vi "Enable-Disable UI by Parameter Sweep.vi"() -> (3 "Controls refs to enable/disable":refnum<vi>[](array[refnum]))   [LabVIEW 2017]
uses:
  Global Variables/gl_UI Ctrl Refs.vi
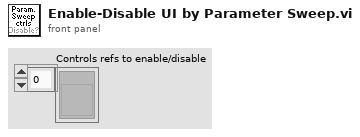
[diagram p1: front panel]
types:
  T1 = typedef "UI ctrl refs cluster.ctl" = cluster{"Top level VI path":path, "Top level VI ref":refnum<vi>, "User menu ref":refnum<k9>, "Sub Panel control":refnum<vi>, "Imaging Param Tab":refnum<vi>, "Occurrence-Start drivers":refnum<k4>, "Occurrence-Speed logging initialised":refnum<k4>, "Occurrence-XYZ stage initialised":refnum<k4>, "Exit button":refnum<vi>, "Status ind":refnum<vi>, "Set as origin":refnum<vi>, "Speed Logging":refnum<vi>, "Time Lapse":refnum<vi>, "Live Imaging":refnum<vi>, "AOL Z Stack":refnum<vi>, "Motor Z Stack":refnum<vi>, "Funct Acq button":refnum<vi>, "Hard Shutter":refnum<vi>, "Virtual Shutter":refnum<vi>, "Laser Power":refnum<vi>, "AOL Mode":refnum<vi>, "Frame Size":refnum<vi>, "Field of View":refnum<vi>, "Dwell Time":refnum<vi>, "Zoom":refnum<vi>, "AOL Z":refnum<vi>, "Objective":refnum<vi>, "Axis":refnum<vi>, "Paths & Names":refnum<vi>, "Experiment folder path (ind.)":refnum<vi>, "Last State (Ind.)":refnum<vi>, "Averages":refnum<vi>, "Angle (degrees)":refnum<vi>, "X centre":refnum<vi>, "Y centre":refnum<vi>, "Plane Mode":refnum<vi>, "# Planes":refnum<vi>, "Z Start":refnum<vi>, "Z Stop":refnum<vi>, "Z Step":refnum<vi>, "PMT 1":refnum<vi>, "PMT 2":refnum<vi>, "Stage XYZ Position":refnum<vi>, "Pockels@Z Start":refnum<vi>, "Pockels@Z Stop":refnum<vi>, "Obtain Z Start":refnum<vi>, "Obtain Z Stop":refnum<vi>, "Live stim.trig.period":refnum<vi>, "Live stim.trig.enable":refnum<vi>, "Movement Correction":refnum<vi>, "Load Reference Image":refnum<vi>, "XY Stage Move":refnum<vi>, "MovCor Cluster":refnum<vi>, "RefDAQParam":refnum<vi>, "Funct. Acq. Pockels Modulation":refnum<vi>, "Ref Laser Power":refnum<vi>, "Enable Video Recording":refnum<vi>, "Video Record-Live Imaging":refnum<vi>, "Video Record-Funct acq":refnum<vi>, "Reference Source":refnum<vi>, "AOL Z-stack Chirps Ready (ind)":refnum<vi>, "Target time between mov.cor. ref triggers (ms)":refnum<vi>, "Funct. Acq. Ref frame save":refnum<vi>, "Tracking button":refnum<vi>, "Show ref plots window":refnum<vi>, "Center freq ind (nm)":refnum<vi>, "Pickup mode (ind)":refnum<vi>, "Logging queue (ind)":refnum<vi>, "Back aperture power (ind.)":refnum<vi>, "Power after objective (ind.)":refnum<vi>, "Switch user":refnum<vi>, "Ls1 Conn. Status":refnum<vi>, "Ls1Tuning Status":refnum<vi>, "Ls1 Faults":refnum<vi>, "Ls1 Connection":refnum<vi>, "Ls1 Mode":refnum<vi>, "Ls1 POWER [mW]":refnum<vi>, "Ls1Shutter":refnum<vi>, "Ls1 Wavelength":refnum<vi>, "Ls1 Note":refnum<vi>, "Ls1 Confirm Wav":refnum<vi>, "Ls1 PreChrp Prism1":refnum<vi>, "Ls1 PreChrp Prism2":refnum<vi>, "Ls1 wav top Ind":refnum<vi>, "Ls1 power top Ind":refnum<vi>, "Ls1 Pump peak Hold":refnum<vi>, "Ls1 Status Ind":refnum<vi>, "Ls1 wav cancel":refnum<vi>, "Experiment Type":refnum<vi>, "Biology Information":refnum<vi>, "Camera recording status":refnum<vi>, "Start Sweep":refnum<vi>, "# Sw. Planes":refnum<vi>}
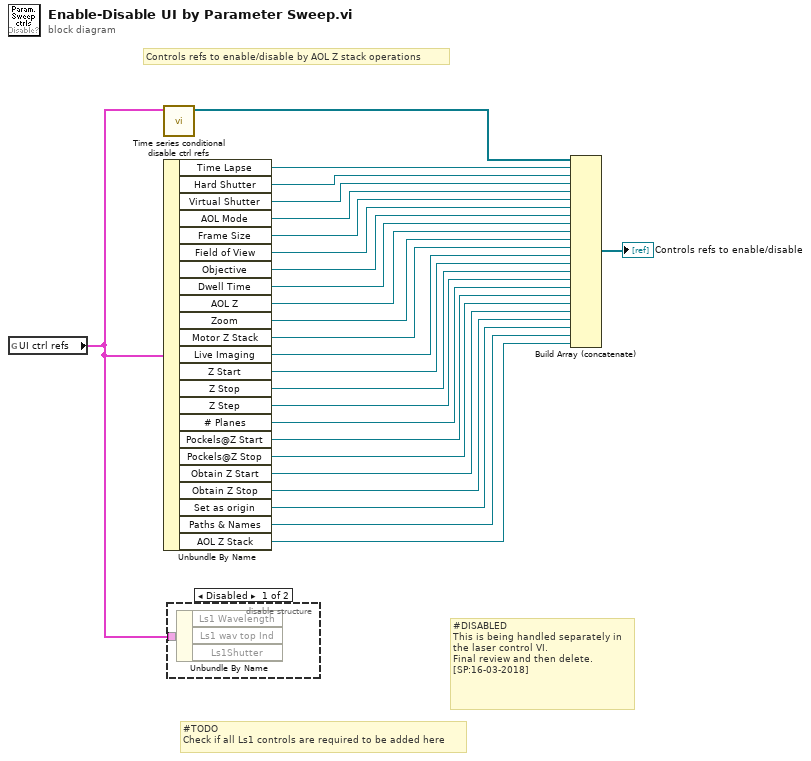
[diagram p0: block diagram]
diagram:
  # "#DISABLED\nThis is being handled separately in\nthe laser control VI.\nFinal review and then delete.\n[SP:16-03-2018]"
  # "#TODO\nCheck if all Ls1 controls are required to be added here"
  # "Controls refs to enable/disable by AOL Z stack operations"
  n1 = global read "gl_UI Ctrl Refs.vi" "UI ctrl refs"() -> (w2:T1)
  n2 = call "Time series conditional disable ctrl refs.vi"("UI ctrl refs"=w2) -> ("Ctrl refs"=w13:refnum<vi>[])  [unwired: 10 in]
  n3 = Unbundle By Name(w2) -> ("Time Lapse"=w26:refnum<vi>, "Hard Shutter"=w22:refnum<vi>, "Virtual Shutter"=w21:refnum<vi>, "AOL Mode"=w20:refnum<vi>, "Frame Size"=w19:refnum<vi>, "Field of View"=w18:refnum<vi>, "Objective"=w17:refnum<vi>, "Dwell Time"=w16:refnum<vi>, "AOL Z"=w15:refnum<vi>, "Zoom"=w14:refnum<vi>, "Motor Z Stack"=w24:refnum<vi>, "Live Imaging"=w25:refnum<vi>, "Z Start"=w12:refnum<vi>, "Z Stop"=w11:refnum<vi>, "Z Step"=w10:refnum<vi>, "# Planes"=w9:refnum<vi>, "Pockels@Z Start"=w8:refnum<vi>, "Pockels@Z Stop"=w7:refnum<vi>, "Obtain Z Start"=w6:refnum<vi>, "Obtain Z Stop"=w5:refnum<vi>, "Set as origin"=w4:refnum<vi>, "Paths & Names"=w3:refnum<vi>, "AOL Z Stack"=w1:refnum<vi>)
  n4 = disable-structure shown="Disabled" {
    disable-tunnel: w2 -> [w27 _]
    frame Disabled {
      n5 = Unbundle By Name(w27) -> ()  [unwired: 3 out]
    }
    frame Enabled {
    }
  }
  n6 = Build Array (concatenate)(w13, w26, w22, w21, w20, w19, w18, w17, w16, w15, w14, w24, w25, w12, w11, w10, w9, w8, w7, w6, w5, w4, w3, w1) -> (→"Controls refs to enable/disable":refnum<vi>[])
